vi "GUI_laptop v11e.vi"() -> ()   [LabVIEW 2019]
uses:
  <vilib>/Math Plots/3D Math Plots/3D Scatter/3D Scatter XCtrl/3D Scatter.xctl
  <vilib>/Platform/TimedLoop/XDataNode/timing_clust.ctl
  <vilib>/Platform/TimedLoop/XDataNode/nitl_modes.ctl
  <vilib>/Platform/TimedLoop/XDataNode/wakeup.ctl
  <vilib>/Analysis/_algsub.llb/Real Vector Norm.vi
  <vilib>/Instr/_visa.llb/VISA Configure Serial Port (Instr).vi
  <vilib>/Utility/file.llb/Write Delimited Spreadsheet (DBL).vi
  <vilib>/addons/System Identification/Data Preprocess.llb/SI Lowpass Filter (MISO Array).vi
  <vilib>/Math Plots/3D Math Plots/3D Scatter/3D Scatter Datatype/Public/Plot Helper (Vector).vi
  <vilib>/platform/TimedLoop/XDataNode/XDataNode.xnode
  <vilib>/Platform/TimedLoop/XDataNode/XDNodeRunTimeDep.lvlib
  <vilib>/Analysis/NI_AALPro.lvlib
  <vilib>/Math Plots/3D Math Plots/3D Scatter/3D Scatter Datatype/3D Scatter Datatype.lvclass
  <vilib>/addons/System Identification/NI_SysID.lvlib
panel:
  in  "Motion scale L1 L2":dbl=10.0
  in  "Motion scale L3":dbl=2.0
  in  "Save Path 4":path=path "C:/Users/jimmy/Documents/GitHub/Arduino-LabVIEW/zhantao/read_data_abs_filtered.csv"
  in  "Save Path 3":path=path "C:/Users/jimmy/Documents/GitHub/Arduino-LabVIEW/zhantao/read_data_abs_sending.csv"
  out "stimulus signals out":dbl[][](array[numeric]) format="%.2f"
  in  "L5 Offset":dbl
  in  "L5 Scale":dbl=1.0
  in  "Motion Scale L4":dbl=2.0
  out "spreadsheet string":string
  in  "Save Path 2":path=path "C:/Users/jimmy/Documents/GitHub/Arduino-LabVIEW/zhantao/read_data_delt.csv"
  out "send values":dbl[](array[numeric])
  out "Robot Feedback (xyz)":dbl[](array[numeric])
  in  "UDP Send":bool
  in  "UDP Recv":bool
  in  "L5 bound":dbl=1000.0
  in  "L4 bound (deg)":dbl=1000.0
  in  "L3 bound (mm)":dbl=1000.0
  in  "L2 bound (deg)":dbl=1000.0
  in  "L1 bound (deg)":dbl=1000.0
  in  "Joystick Type":dbl(ring) items=["Rigid Joystick", "Free Joystick"]
  out "Finished Late? [i-1]":bool
  in  "Epsilon":dbl=0.2
  out "3D Scatter":refnum<class "3D Plot Datatype.lvclass">[](xcontrol)
  out "Random Point":dbl[](array[numeric])
  out "Virtual Cursor":dbl[](array[numeric])
  out "Iteration Duration":i64
  in  "Num of Points":i32=10
  in  "z bound":dbl=2.0
  in  "y bound":dbl=5.0
  in  "x bound":dbl=5.0
  in  "Stop":bool
  in  "Round Decimals":dbl=2.0 format="%#_15g"
  in  "Save  Data":bool
  in  "Save Path":path=path "C:/Users/jimmy/Documents/GitHub/Arduino-LabVIEW/zhantao/read_data_abs.csv"
  in  "x speed":dbl=0.5
  in  "z speed":dbl=0.5
  in  "y speed":dbl=0.5
  out "error out":errorcluster
  in  "baud rate":u32=115200
  in  "VISA resource name":refnum<visa-resource-name>
  # "Joystick Selection"
  # "Plotting"
  # "Data Saving"
  # "Arduino Communication"
  # "Master Slave Communication"
  # "Parameters"
  # "TODO: fix the bounds; currently bounds are arbitrary"
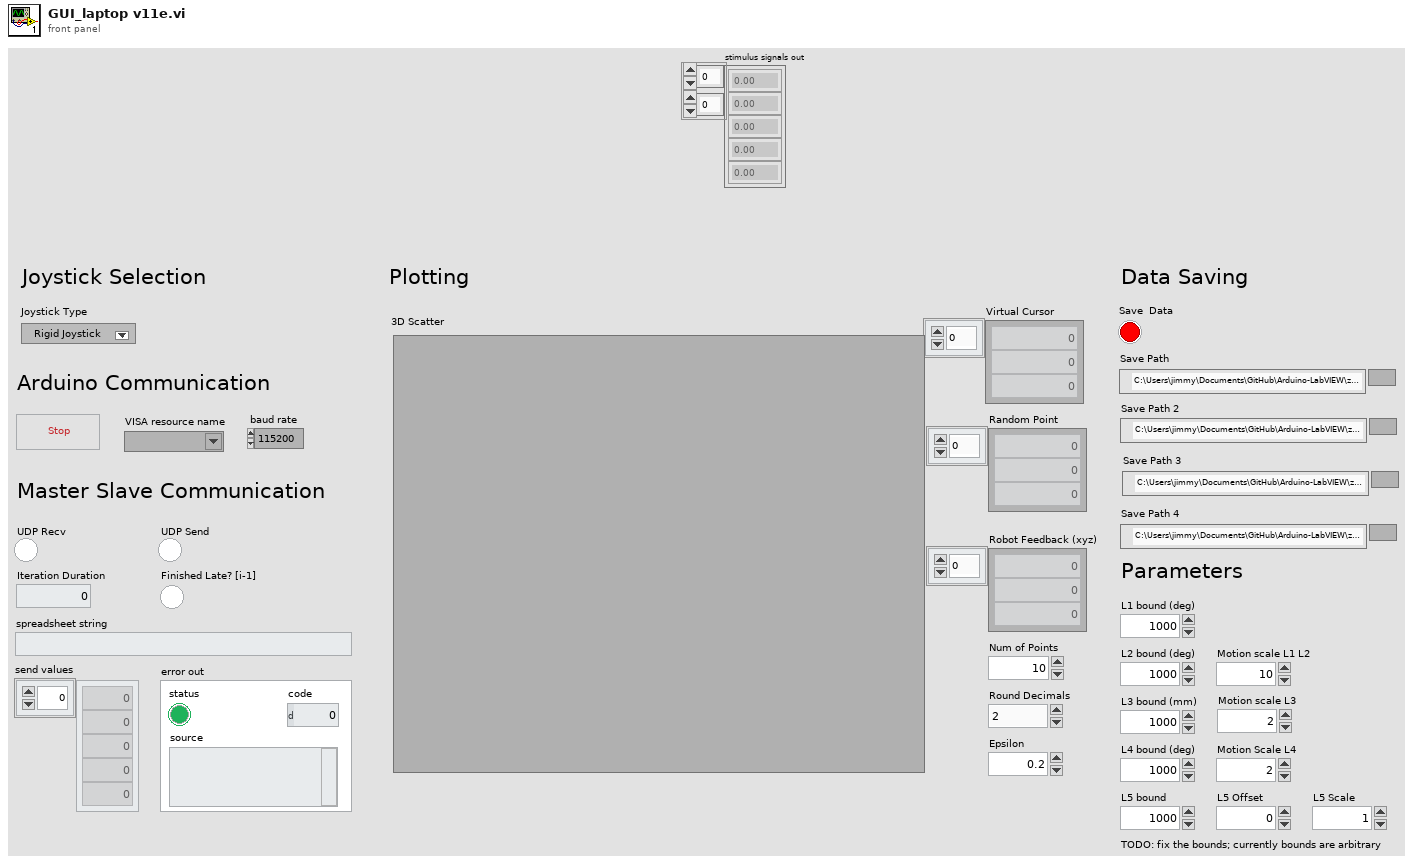
[diagram p1: front panel]
types:
  T1 = typedef "XDNodeRunTimeDep.lvlib/timing_clust.ctl" = cluster{"Expected End [f-1]":u64, "Actual End [f-1]":u64, "Finished Late? [f-1]":bool, "Expected End [i-1]":u64, "Actual End [i-1]":u64, "Finished Late? [i-1]":bool, "Expected Start [i]":u64, "Actual Start [i]":u64, "Expected Start [f]":u64, "Actual Start [f]":u64, "Source Name":string, "Structure Name":string, "Period":i64, "Deadline":i64, "Offset":i64, "Start":i64, "Priority":i32, "Timeout":i32, "Mode":T2, "Wakeup Reason":T3, "Error":errorcluster, "Source Type":string, "Secondary Source Type":string, "Global End Time":u64, "Global Start Time":u64, "Frame Duration":u64, "Iteration Duration":u64, "Assigned CPU":i32, "I/O Scan Engine Mode":u32}
  T2 = typedef "XDNodeRunTimeDep.lvlib/nitl_modes.ctl" = enum32{"No Change", "Process missed periods, maintain original phase", "Discard missed periods, maintain original phase", "Process missed periods, ignore original phase", "Discard missed periods, ignore original phase"}
  T3 = typedef "XDNodeRunTimeDep.lvlib/wakeup.ctl" = enum32{"Normal", "Aborted", "Asynchronous wakeup", "Timing source error", "Timed loop error", "Timeout"}
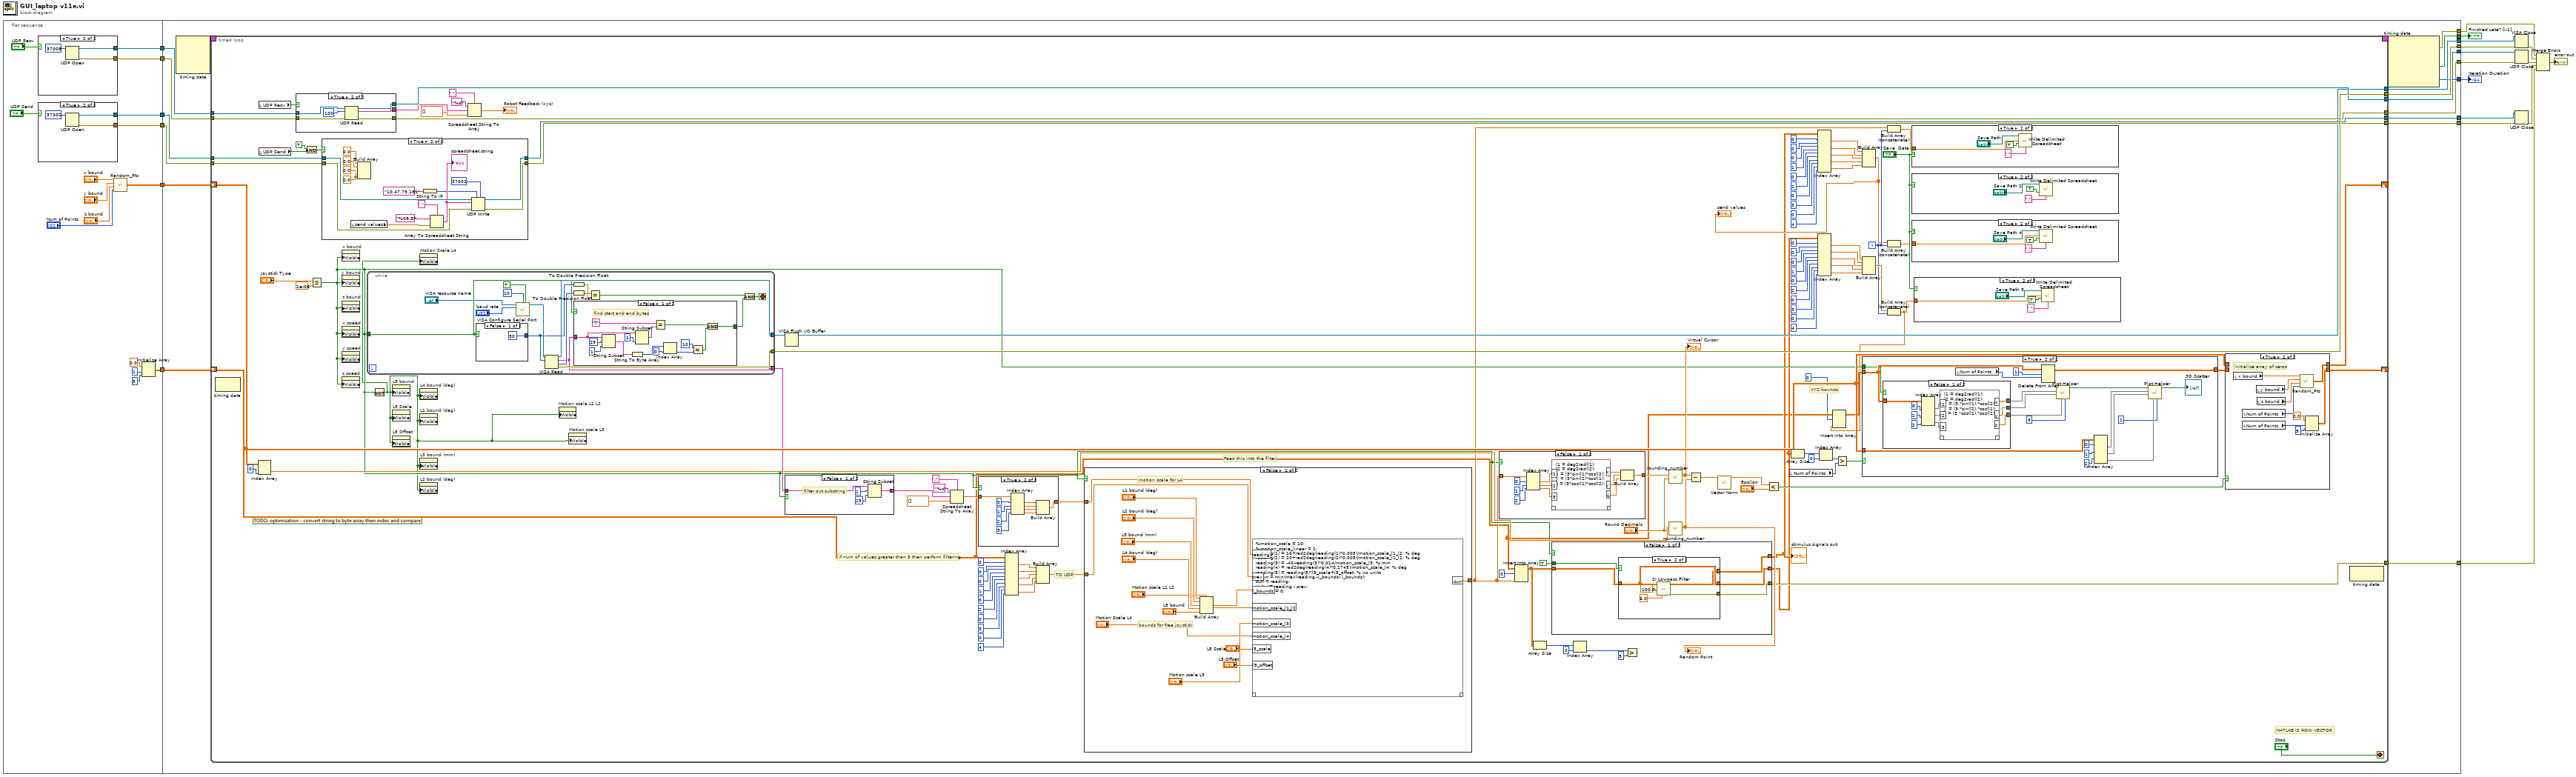
[diagram p0: block diagram]
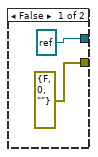
[diagram p2: hidden frame]
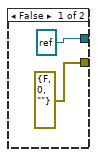
[diagram p3: hidden frame]
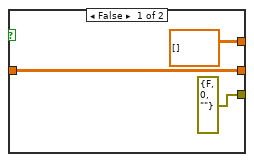
[diagram p6: hidden frame]
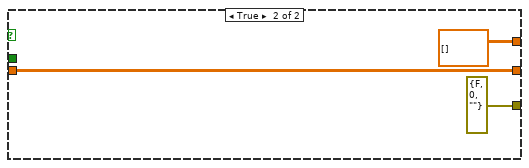
[diagram p7: hidden frame]
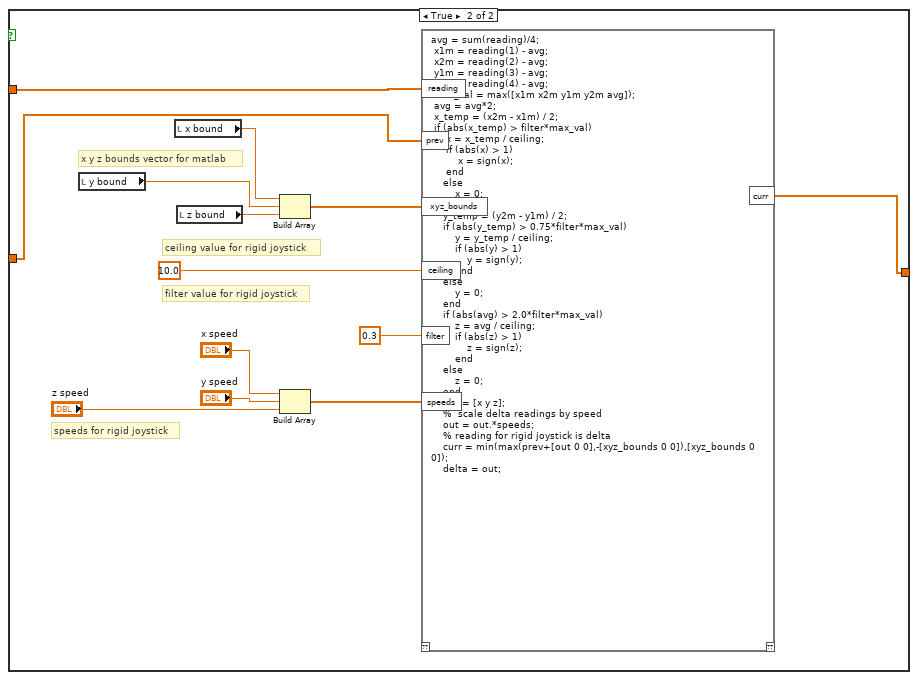
[diagram p8: hidden frame]
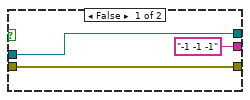
[diagram p11: hidden frame]
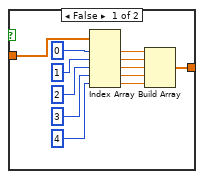
[diagram p15: hidden frame]
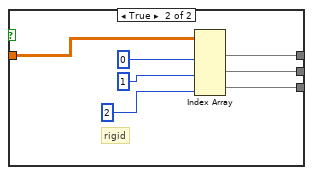
[diagram p18: hidden frame]
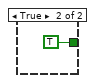
[diagram p19: hidden frame]
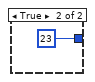
[diagram p20: hidden frame]
diagram:
  n1 = flat-sequence {
    tunnel: [w27] -> w16
    tunnel: [w31] -> w15
    tunnel: [w26] -> w14
    tunnel: [w25] -> w13
    tunnel: [w22] -> w12
    tunnel: [w21] -> w11
    tunnel: [w61] -> w20
    tunnel: [w60] -> w19
    tunnel: [w58] -> w10
    tunnel: [w56] -> w18
    tunnel: [w55] -> w17
    tunnel: w16 -> [w59]
    tunnel: w15 -> [w57]
    tunnel: w14 -> [w54]
    tunnel: w13 -> [w53]
    tunnel: w12 -> [w52]
    tunnel: w11 -> [w51]
    tunnel: [w50] -> w4
    tunnel: [w49] -> w9
    tunnel: [w48] -> w3
    tunnel: [w47] -> w2
    tunnel: [w46] -> w1
    frame #0 {
      n2 = case shown="True" "UDP Recv" {
        tunnel: [refnum<k16> refnum ("port") w44] -> w25
        tunnel: [errorcluster {"status"=FALSE, "code"=0, "source"=""} ("error out") w43] -> w22
        frame False {
        }
        frame True {
          n3 = UDP Open(11:u16 37008 ("port")) -> (port=w44:refnum<k16>, 0:w43:errorcluster)  [unwired: 4 in, 1 out]
        }
      }
      n4 = case shown="True" "UDP Send" {
        tunnel: [refnum<k16> refnum ("port") w39] -> w26
        tunnel: [errorcluster {"status"=FALSE, "code"=0, "source"=""} ("error out") w38] -> w21
        frame False {
        }
        frame True {
          n5 = UDP Open(11:u16 37002 ("port")) -> (port=w39:refnum<k16>, 0:w38:errorcluster)  [unwired: 4 in, 1 out]
        }
      }
      n6 = call "Random_Pts.vi"("Num of Points"="Num of Points", "z bound"="z bound", "y bound"="y bound", "x bound"="x bound") -> ("appended array"=w31:dbl[][])
      n7 = Initialize Array(0.0 ("element"), 1 ("dimension size"), 5 ("dimension size")) -> (w27:dbl[][])
    }
    frame #1 {
      n8 = node-c288() -> (w63:T1)  [unwired: 4 in]
      n9 = timed-loop {
        tunnel: [w121] -> w61
        tunnel: [w180] -> w60
        shift-right: [w179] -> _
        shift-left: w59 -> [w69]
        timing: w63 -> [_]
        timing-out: [_] -> w62
        shift-right: [w175] -> _
        shift-left: w57 -> [w176]
        tunnel: w54 -> [w138]
        tunnel: w53 -> [w137]
        tunnel: w52 -> [w135]
        tunnel: w51 -> [w134]
        tunnel: [w133] -> w50
        tunnel: [w132] -> w49
        tunnel: [w131] -> w48
        tunnel: [w130] -> w47
        tunnel: [w109] -> w46
        i -> [w73]
        stop <- "Stop" stop-if-true
        # "XYZ bounds"
        # "if num of values greater than 5 then perform filtering"
        # "Feed this into the filter"
        # "TO UDP"
        # "MATLAB IS ROW VECTOR"
        n10 = node-c288() -> ()  [unwired: 1 in, 1 out]
        n11 = Index Array(array=w176, index (col)=0 ("index (row)")) -> (element=w147:dbl[])  [unwired: 1 in]
        n12 = local read "UDP Recv"() -> (w136:bool)
        n13 = local read "UDP Send"() -> (w124:bool)
        n14 = case shown="True" w136 {
          tunnel: w137 -> [w254 w261]
          tunnel: w135 -> [w255 w260]
          tunnel: [w255 w259] -> w133
          tunnel: [w254 w258] -> w131
          tunnel: ["-1 -1 -1" w256] -> w126
          frame False {
          }
          frame True {
            n15 = UDP Read(connection ID=w261, max size (548)=100, 8:w260) -> (data out=w256:string, error out=w259:errorcluster, 3:w258:refnum<k16>)  [unwired: 1 in, 2 out]
          }
        }
        n16 = And(x=TRUE, y=w124) -> (x .and. y?=w123:bool)
        n17 = Less Or Equal?(x="Joystick Type", y=1e-06) -> (x <= y?=w110:bool)
        n18 = case shown="True" w123 {
          tunnel: w138 -> [w236 w252]
          tunnel: w134 -> [w237 w248]
          tunnel: [w237 w244] -> w132
          tunnel: [w236 w243] -> w130
          frame False {
          }
          frame True {
            w242 = 0.0 ("element")
            n19 = local read "send values"() -> (w238:dbl[])
            n20 = Build Array(0.0 ("element"), 0.0 ("element"), 0.0 ("element"), w242, w242) -> ()  [unwired: 1 out]
            n21 = String To IP(1:"10.47.79.181" ("name")) -> (0:w246:u32)
            n22 = Array To Spreadsheet String(delimiter (Tab)=" ", array=w238, 3:"%08.3f" ("format string")) -> (spreadsheet string=w249:string)
            "spreadsheet string" <- w249
            n23 = UDP Write(address=w246, port or service name=u16 37001, connection ID=w252, data in=w249, 8:w248) -> (error out=w244:errorcluster, 3:w243:refnum<k16>)  [unwired: 1 in]
          }
        }
        n24 = property on="x bound" class="DigNum (strict)"("Visible"=w110) -> ()  [unwired: 2 in, 2 out]
        n25 = property on="y bound" class="DigNum (strict)"("Visible"=w110) -> ()  [unwired: 2 in, 2 out]
        n26 = property on="z bound" class="DigNum (strict)"("Visible"=w110) -> ()  [unwired: 2 in, 2 out]
        n27 = property on="x speed" class="DigNum (strict)"("Visible"=w110) -> ()  [unwired: 2 in, 2 out]
        n28 = property on="y speed" class="DigNum (strict)"("Visible"=w110) -> ()  [unwired: 2 in, 2 out]
        n29 = property on="z speed" class="DigNum (strict)"("Visible"=w110) -> ()  [unwired: 2 in, 2 out]
        n30 = while {
          tunnel: [w353] -> w149
          tunnel: [w366] -> w180
          tunnel: [w360] -> w122
          tunnel: w110 -> [w354]
          stop <- w356 stop-if-true
          n31 = case shown="False" w354 {
            tunnel: [30 u32 23 ("byte count")] -> w359
            frame False {
            }
            frame True {
            }
          }
          n32 = call-poly "VISA Configure Serial Port"("VISA resource name"="VISA resource name", "termination char\n(0xA = '\\n' = LF)"=u8 10 ("termination char\n(0xA = '\\n' = LF)"), "Enable Termination\nChar (T)"=TRUE ("Enable Termination\nChar (T)"), "baud rate (9600)"="baud rate") -> ("VISA resource name out"=w361:refnum<visa-resource-name>)  [unwired: 10 in, 1 out]
          n33 = VISA Read(VISA resource name=w361, byte count=w359) -> (VISA resource name out=w360:refnum<visa-resource-name>, read buffer=w353:string, return count=w368:u32, error out=w366:errorcluster)  [unwired: 1 in]
          n34 = To Double Precision Float(number=w359) -> (double precision float=w358:dbl)
          n35 = To Double Precision Float(number=w368) -> (double precision float=w367:dbl)
          n36 = case shown="False" w354 {
            tunnel: [w375 TRUE] -> w355
            tunnel: w353 -> [w378 _]
            frame False {
              # "find start and end bytes"
              n37 = String Subset(string=w378, offset (0)=29, length (rest)=1) -> (substring=w373:string)
              n38 = String To Byte Array(string=w373) -> (unsigned byte array=w372:u8[])
              n39 = String Subset(string=w378, length (rest)=1) -> (substring=w381:string)  [unwired: 1 in]
              n40 = Equal?(x="T", y=w381) -> (x = y?=w377:bool)
              n41 = Index Array(array=w372, index=0) -> (element=w370:u8)
              n42 = Equal?(x=10, y=w370) -> (x = y?=w376:bool)
              n43 = And(x=w377, y=w376) -> (x .and. y?=w375:bool)
            }
            frame True {
            }
          }
          n44 = Equal?(x=w367, y=w358) -> (x = y?=w357:bool)
          n45 = And(x=w357, y=w355) -> (x .and. y?=w356:bool)
        }
        n46 = Not(x=w110) -> (.not. x?=w64:bool)
        n47 = property on="L5 bound" class="DigNum (strict)"("Visible"=w64) -> ()  [unwired: 2 in, 2 out]
        n48 = property on="L5 Scale" class="DigNum (strict)"("Visible"=w64) -> ()  [unwired: 2 in, 2 out]
        n49 = property on="L5 Offset" class="DigNum (strict)"("Visible"=w64) -> ()  [unwired: 2 in, 2 out]
        n50 = property on="Motion Scale L4" class="DigNum (strict)"("Visible"=w64) -> ()  [unwired: 2 in, 2 out]
        n51 = property on="L4 bound (deg)" class="DigNum (strict)"("Visible"=w64) -> ()  [unwired: 2 in, 2 out]
        n52 = property on="L1 bound (deg)" class="DigNum (strict)"("Visible"=w64) -> ()  [unwired: 2 in, 2 out]
        n53 = property on="L3 bound (mm)" class="DigNum (strict)"("Visible"=w64) -> ()  [unwired: 2 in, 2 out]
        n54 = property on="L2 bound (deg)" class="DigNum (strict)"("Visible"=w64) -> ()  [unwired: 2 in, 2 out]
        n55 = Spreadsheet String To Array(delimiter (Tab)=" ", format string="%d", spreadsheet string=w126, array type (2D Dbl)=dbl[] []) -> (array=→"Robot Feedback (xyz)":dbl[])
        n56 = property on="Motion scale L1 L2" class="DigNum (strict)"("Visible"=w64) -> ()  [unwired: 2 in, 2 out]
        n57 = property on="Motion scale L3" class="DigNum (strict)"("Visible"=w64) -> ()  [unwired: 2 in, 2 out]
        n58 = VISA Flush I/O Buffer(VISA resource name=w122) -> (VISA resource name out=w121:refnum<visa-resource-name>)  [unwired: 2 in, 1 out]
        n59 = case shown="False" w110 {
          tunnel: w149 -> [w280 w281]
          tunnel: [w277 w281] -> w148
          frame False {
            # "filter out substring"
            n60 = String Subset(string=w280, offset (0)=1, length (rest)=29) -> (substring=w277:string)
          }
          frame True {
          }
        }
        n61 = Spreadsheet String To Array(delimiter (Tab)=",", format string="%d", spreadsheet string=w148, array type (2D Dbl)=dbl[] []) -> (array=w150:dbl[])
        n62 = case shown="True" w110 {
          tunnel: w150 -> [w282 w297]
          tunnel: [w287 w296] -> w118
          frame False {
            n63 = Index Array(array=w282, index #1=0 ("Plot ID"), index #2=1 ("Plot ID"), index #3=2 ("Plot ID"), index #4=3 ("Plot ID"), index #5=4 ("Plot ID")) -> (element #1=w290:dbl, element #2=w289:dbl, element #3=w288:dbl, element #4=w284:dbl, element #5=w283:dbl)
            n64 = Build Array(w290, w289, w288, w284, w283) -> (w287:dbl[])
          }
          frame True {
            n65 = Index Array(array=w297, index #1=0 ("Plot ID"), index #2=1 ("Plot ID"), index #3=2 ("Plot ID"), index #4=3 ("index")) -> (element #1=w300:dbl, element #2=w299:dbl, element #3=w298:dbl, element #4=w294:dbl)
            n66 = Build Array(w300, w299, w298, w294) -> (w296:dbl[])
          }
        }
        n67 = Index Array(array=w69, index (row) #1=0 ("disabled index (row)"), index (col) #1=0 ("disabled index (col)"), index (row) #2=0 ("disabled index (row)"), index (col) #2=1 ("disabled index (col)"), index (row) #3=0 ("disabled index (row)"), index (col) #3=2 ("disabled index (col)"), index (row) #4=0 ("disabled index (row)"), index (col) #4=3 ("disabled index (col)"), index (row) #5=0 ("disabled index (row)"), index (col) #5=4 ("disabled index (col)")) -> (element #1=w161:dbl, element #2=w160:dbl, element #3=w159:dbl, element #4=w152:dbl, element #5=w151:dbl)
        n68 = Build Array(w161, w160, w159, w152, w151) -> (w119:dbl[])
        n69 = case shown="False" w110 {
          tunnel: w119 -> [w211 w222]
          tunnel: w118 -> [w212 w221]
          tunnel: [w210 w220] -> w93
          frame False {
            # "bounds for free joystick"
            # "motion scale for L4"
            n70 = Build Array("L1 bound (deg)", "L2 bound (deg)", "L3 bound (mm)", "L4 bound (deg)", "L5 bound") -> (w213:dbl[])
            n71 = script code="%motion_scale = 10;\n%motion_scale_linear = 2;\nreading(1) = 16+rad2deg(reading(1)*0.005)/motion_scale_l1_l2; % deg\nreading(2) = 20+rad2deg(reading(2)*0.005)/motion_scale_l1_l2; % deg\nreading(3) = -40-reading(3)*0.014/motion_scale_l3; % mm\nreading(4) = rad2deg(reading(4)*0.1745)/motion_scale_l4; % deg\nreading(5) = reading(5)*l5_scale+l5_offset; % no units\n%curr = min(max(reading,-l_bounds),l_bounds);\ncurr = reading;\ndelta = reading - prev;\ndelta(5) = 0;"("l_bounds"=w213, "motion_scale_l4"="Motion Scale L4", "reading"=w212, "prev"=w211, "l5_scale"="L5 Scale", "l5_offset"="L5 Offset", "motion_scale_l3"="Motion scale L3", "motion_scale_l1_l2"="Motion scale L1 L2") -> ("curr"=w210:dbl[])  [unwired: 1 in, 1 out]
          }
          frame True {
            # "ceiling value for rigid joystick"
            # "filter value for rigid joystick"
            # "speeds for rigid joystick"
            # "x y z bounds vector for matlab"
            n72 = local read "y bound"() -> (w231:dbl)
            n73 = local read "x bound"() -> (w230:dbl)
            n74 = local read "z bound"() -> (w232:dbl)
            n75 = Build Array(w230, w231, w232) -> (w223:dbl[])
            n76 = Build Array("x speed", "y speed", "z speed") -> (w226:dbl[])
            n77 = script code="avg = sum(reading)/4;\n x1m = reading(1) - avg;\n x2m = reading(2) - avg;\n y1m = reading(3) - avg;\n y2m = reading(4) - avg;\n max_val = max([x1m x2m y1m y2m avg]);\n avg = avg*2;\n x_temp = (x2m - x1m) / 2;\n if (abs(x_temp) > filter*max_val)\n     x = x_temp / ceiling;\n     if (abs(x) > 1)\n         x = sign(x);\n     end\n    else\n        x = 0;\n    end\n    y_temp = (y2m - y1m) / 2;\n    if (abs(y_temp) > 0.75*filter*max_val)\n        y = y_temp / ceiling;\n        if (abs(y) > 1)\n            y = sign(y);\n        end\n    else\n        y = 0;\n    end\n    if (abs(avg) > 2.0*filter*max_val)\n        z = avg / ceiling;\n        if (abs(z) > 1)\n            z = sign(z);\n        end\n    else\n        z = 0;\n    end\n    out = [x y z];\n    %  scale delta readings by speed\n    out = out.*speeds;\n    % reading for rigid joystick is delta\n    curr = min(max(prev+[out 0 0],-[xyz_bounds 0 0]),[xyz_bounds 0 0]);\n    delta = out;"("xyz_bounds"=w223, "ceiling"=10.0 ("Real"), "filter"=0.3 ("Real"), "speeds"=w226, "reading"=w221, "prev"=w222) -> ("curr"=w220:dbl[])  [unwired: 1 in, 1 out]
          }
        }
        n78 = case shown="False" w110 {
          tunnel: [w308 w315] -> w177
          tunnel: w93 -> [w307 w315]
          frame False {
            n79 = Index Array(array=w307, index #1=0 ("Plot ID"), index #2=1 ("Plot ID"), index #3=2 ("Plot ID")) -> (element #1=w306:dbl, element #2=w305:dbl, element #3=w304:dbl)
            n80 = script code="l1 = deg2rad(l1);\nl2 = deg2rad(l2);\nx = l3*sin(l1)*cos(l2);\ny = l3*sin(l2)*cos(l1);\nz = l3*cos(l1)*cos(l2);"("l1"=w306, "l2"=w305, "l3"=w304) -> ("x"=w311:dbl, "y"=w310:dbl, "z"=w309:dbl)  [unwired: 1 in, 1 out]
            n81 = Build Array(w311, w310, w309) -> (w308:dbl[])
          }
          frame True {
          }
        }
        n82 = Insert Into Array(array=w69, index (row)=0, new element=w93) -> (w111:dbl[][])  [unwired: 1 in]
        n83 = Array Size(array=w111) -> (size(s)=w114:i32[])
        n84 = case shown="False" w110 {
          tunnel: TRUE -> [w192 _]
          tunnel: w111 -> [w194 w205]
          tunnel: [w193 w205] -> w70
          tunnel: [w191 errorcluster {"status"=FALSE, "code"=0, "source"=""} ("error out")] -> w109
          tunnel: [w190 dbl[][] [] ("stimulus signals out")] -> w71
          frame False {
            n85 = case shown="True" w192 {
              tunnel: w194 -> [w197 w199]
              tunnel: [w197 w199] -> w193
              tunnel: [errorcluster {"status"=FALSE, "code"=0, "source"=""} ("error out") w200] -> w191
              tunnel: [dbl[][] [] ("stimulus signals out") w198] -> w190
              frame False {
              }
              frame True {
                n86 = call-poly <vilib>:"SI Lowpass Filter.vi"("cutoff frequency"=6.0, "sampling rate (Hz)"=100.0, "stimulus signals in"=w199) -> ("error out"=w200:errorcluster, "stimulus signals out"=w198:dbl[][])  [unwired: 6 in, 1 out]
              }
            }
          }
          frame True {
          }
        }
        "stimulus signals out" <- w71
        n87 = Index Array(array=w114, index=0) -> (element=w113:i32)
        n88 = Greater?(x=w113, y=5) -> ()  [unwired: 1 out]
        n89 = call "rounding_number.vi"("power of ten"="Round Decimals", "Array"=w177) -> ("rounded"=w145:dbl[])  [unwired: 9 in]
        "Virtual Cursor" <- w145
        n90 = call "rounding_number.vi"("power of ten"="Round Decimals", "Array"=w147) -> ("rounded"=w144:dbl[])  [unwired: 9 in]
        "Random Point" <- w144
        n91 = Subtract(x=w145, y=w144) -> (x-y=w143:dbl[])
        n92 = call-poly <vilib>:"Vector Norm.vi"("Input Vector"=w143) -> ("norm"=w142:dbl)  [unwired: 9 in, 1 out]
        n93 = Less?(x=w142, y="Epsilon") -> (x < y?=w140:bool)
        n94 = local read "Num of Points"() -> (w163:i32)
        n95 = Array Size(array=w70) -> (size(s)=w117:i32[])
        n96 = Index Array(array=w71, index (row) #1=0 ("disabled index (col)"), index (col) #1=0 ("disabled index (row)"), index (row) #2=0 ("disabled index (col)"), index (col) #2=1 ("disabled index (row)"), index (row) #3=0 ("disabled index (col)"), index (col) #3=2 ("disabled index (row)"), index (row) #4=0 ("disabled index (col)"), index (col) #4=3 ("disabled index (row)"), index (row) #5=0 ("disabled index (col)"), index (col) #5=4 ("disabled index (col)")) -> (element #1=w79:dbl, element #2=w78:dbl, element #3=w77:dbl, element #4=w76:dbl, element #5=w75:dbl)
        n97 = Index Array(array=w70, index (row) #1=0 ("disabled index (col)"), index (col) #1=0 ("disabled index (row)"), index (row) #2=0 ("disabled index (col)"), index (col) #2=1 ("disabled index (row)"), index (row) #3=0 ("disabled index (col)"), index (col) #3=2 ("disabled index (row)"), index (row) #4=0 ("disabled index (col)"), index (col) #4=3 ("disabled index (row)"), index (row) #5=0 ("disabled index (col)"), index (col) #5=4 ("disabled index (col)")) -> (element #1=w98:dbl, element #2=w97:dbl, element #3=w96:dbl, element #4=w95:dbl, element #5=w94:dbl)
        n98 = Index Array(array=w117, index=0) -> (element=w164:i32)
        n99 = Greater?(x=w164, y=w163) -> (0:w162:bool)
        n100 = Build Array(w79, w78, w77, w76, w75) -> (w72:dbl[])
        "send values" <- w72
        n101 = Build Array(w98, w97, w96, w95, w94) -> (w91:dbl[])
        n102 = Build Array (concatenate)(w93, w73) -> (w92:dbl[])
        n103 = Build Array (concatenate)(w72, w73) -> (w67:dbl[])
        n104 = Build Array (concatenate)(w91, w73) -> (w65:dbl[])
        n105 = Insert Into Array(array=w69, index (row)=0, new element=w65) -> (w66:dbl[][])  [unwired: 1 in]
        n106 = case shown="True" w162 {
          tunnel: w66 -> [w316 w334]
          tunnel: [w316 w333] -> w178
          tunnel: w176 -> [_ w332]
          tunnel: w110 -> [_ w317]
          frame False {
          }
          frame True {
            n107 = case shown="False" w317 {
              tunnel: w334 -> [w345 w349]
              tunnel: [w336 w348] -> w323
              tunnel: [w337 w347] -> w322
              tunnel: [w338 w346] -> w321
              frame False {
                n108 = Index Array(array=w345, index (col) #1=0 ("Plot ID"), index (col) #2=1 ("Plot ID"), index (col) #3=2 ("Plot ID")) -> (element #1=w341:dbl[], element #2=w340:dbl[], element #3=w339:dbl[])  [unwired: 3 in]
                n109 = script code="l1 = deg2rad(l1);\nl2 = deg2rad(l2);\nx = l3.*sin(l1).*cos(l2);\ny = l3.*sin(l2).*cos(l1);\nz = l3.*cos(l1).*cos(l2);"("l1"=w341, "l2"=w340, "l3"=w339) -> ("x"=w336:dbl[], "y"=w337:dbl[], "z"=w338:dbl[])  [unwired: 1 in, 1 out]
              }
              frame True {
                # "rigid"
                n110 = Index Array(array=w349, index (col) #1=0 ("disabled index (col)"), index (col) #2=1 ("index (col)"), index (col) #3=2 ("index (col)")) -> (element #1=w348:dbl[], element #2=w347:dbl[], element #3=w346:dbl[])  [unwired: 3 in]
              }
            }
            n111 = local read "Num of Points"() -> (w331:i32)
            n112 = Delete From Array(array=w334, length=1, index (row)=w331) -> (array with subset deleted=w333:dbl[][])  [unwired: 1 in, 1 out]
            n113 = call-poly <vilib>:"Plot Helper.vi"("Plot ID"=0, "z vector"=w321, "y vector"=w322, "x vector"=w323) -> ("3D Plot lvclass Array out"=w325:refnum<class "3D Plot Datatype.lvclass">[])  [unwired: 2 in, 5 out]
            n114 = Index Array(array=w332, index (row) #1=0 ("index (row)"), index (row) #2=1 ("index (row)"), index (row) #3=2 ("index (row)")) -> (element #1=w329:dbl[], element #2=w328:dbl[], element #3=w327:dbl[])  [unwired: 3 in]
            n115 = call-poly <vilib>:"Plot Helper.vi"("Plot ID"=1, "z vector"=w327, "y vector"=w328, "x vector"=w329, "3D Plot lvclass Array in"=w325) -> ("3D Plot lvclass Array out"=→"3D Scatter":refnum<class "3D Plot Datatype.lvclass">[])  [unwired: 1 in, 5 out]
          }
        }
        n116 = case shown="True" "Save  Data" {
          tunnel: w92 -> [_ w262]
          frame False {
          }
          frame True {
            n117 = call-poly <vilib>:"Write Delimited Spreadsheet.vi"("file path (dialog if empty)"="Save Path", "1D data"=w262, "append to file? (new file:F)"=TRUE, "delimiter (\\t)"="," ("delimiter (\\t)")) -> ()  [unwired: 10 in, 2 out]
          }
        }
        n118 = case shown="True" "Save  Data" {
          frame False {
          }
          frame True {
            n119 = call-poly <vilib>:"Write Delimited Spreadsheet.vi"("file path (dialog if empty)"="Save Path 2", "append to file? (new file:F)"=TRUE, "delimiter (\\t)"="," ("delimiter (\\t)")) -> ()  [unwired: 11 in, 2 out]
          }
        }
        n120 = case shown="True" "Save  Data" {
          tunnel: w67 -> [_ w182]
          frame False {
          }
          frame True {
            n121 = call-poly <vilib>:"Write Delimited Spreadsheet.vi"("file path (dialog if empty)"="Save Path 4", "1D data"=w182, "append to file? (new file:F)"=TRUE, "delimiter (\\t)"="," ("delimiter (\\t)")) -> ()  [unwired: 10 in, 2 out]
          }
        }
        n122 = case shown="True" "Save  Data" {
          tunnel: w65 -> [_ w186]
          frame False {
          }
          frame True {
            n123 = call-poly <vilib>:"Write Delimited Spreadsheet.vi"("file path (dialog if empty)"="Save Path 3", "1D data"=w186, "append to file? (new file:F)"=TRUE, "delimiter (\\t)"="," ("delimiter (\\t)")) -> ()  [unwired: 10 in, 2 out]
          }
        }
        n124 = case shown="True" w140 {
          tunnel: w176 -> [w267 _]
          tunnel: [w267 w272] -> w175
          tunnel: w178 -> [w266 _]
          tunnel: [w266 w268] -> w179
          frame False {
          }
          frame True {
            # "initialize array of zeros"
            n125 = local read "x bound"() -> (w276:dbl)
            n126 = local read "Num of Points"() -> (w273:i32)
            n127 = local read "Num of Points"() -> (w270:i32)
            n128 = local read "y bound"() -> (w275:dbl)
            n129 = local read "z bound"() -> (w274:dbl)
            n130 = call "Random_Pts.vi"("Num of Points"=w273, "z bound"=w274, "y bound"=w275, "x bound"=w276) -> ("appended array"=w272:dbl[][])
            n131 = Initialize Array(0.0 ("element"), w270, 5 ("dimension size")) -> (w268:dbl[][])
          }
        }
        n132 = node-c288() -> ()  [unwired: 1 in, 1 out]
      }
      n133 = node-c288(w62) -> (w58:errorcluster, w55:bool, w56:i64)  [unwired: 3 out]
    }
  }
  n134 = VISA Close(VISA resource name=w20, error in (no error)=w19) -> (error out=w8:errorcluster)
  n135 = UDP Close(connection ID=w3, 8:w4) -> (error out=w7:errorcluster)  [unwired: 1 out]
  n136 = UDP Close(connection ID=w2, 8:w9) -> (error out=w6:errorcluster)  [unwired: 1 out]
  n137 = Merge Errors(w10, w8, w7, w6, w1) -> (→"error out":errorcluster)
  "Iteration Duration" <- w18
  "Finished Late? [i-1]" <- w17
